vi "13.4.1 Realworld Particle.vi"(8 "ErrI":errorcluster) -> (0 "ErrO":errorcluster)   [LabVIEW 2016]
uses:
  <vilib>/vision/Image Controls.llb/IMAQ Image.ctl
  <vilib>/vision/Calibration.llb/Distortion Model.ctl
  <vilib>/vision/Calibration.llb/Distortion Model Types.ctl
  <vilib>/vision/Measure.llb/Edge Options.ctl
  <vilib>/vision/Measure.llb/Edge Polarity.ctl
  <vilib>/vision/NI_Vision_Development_Module.lvlib
panel:
  out "Center of Mass of Holes\n(mm, x and y to orign)":dbl[][](array[numeric]) format="%.2f"
  out "Image":T1(plugin-control)
  in  "Next":bool
  in  "Exit":bool
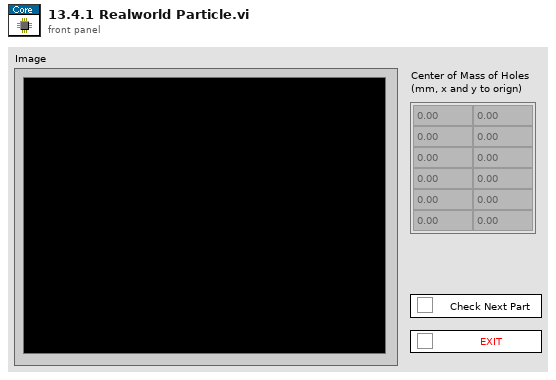
[diagram p1: front panel]
types:
  T1 = typedef "IMAQ Image.ctl" = refnum<image>
  T2 = typedef "Distortion Model.ctl" = cluster{"Distortion Model":T3, "Polynomial Model Setup":cluster{"Radial Coefficient":u32, "Tangential Coefficients ":bool}}
  T3 = typedef "Distortion Model Types.ctl" = i32
  T4 = typedef "Edge Options.ctl" = cluster{"Edge Polarity":T5, "Kernel Size":u32, "Width":u32, "Minimum Edge Strength":sgl, "Interpolation Type":enum32{"Zero Order", "Bilinear", "Quadratic", "Cubic", "Bilinear Fixed"}, "Data Processing Method":enum32{"Average", "Median"}}
  T5 = typedef "Edge Polarity.ctl" = u32
  T6 = cluster{"Direction":u16, "Primary Edge Options":T4, "Secondary Edge Options":T4, "Show Search Area":bool, "Show Search Lines":bool, "Show Edges Found":bool, "Show Result":bool, "Search Area Color":u32, "Search Lines Color":u32, "Edge Locations Color":u32, "Result Color":u32, "Overlay Group Name":string}
  T7 = typedef "IMAQ Rectangle" = cluster{"Left":i32, "Top":i32, "Right":i32, "Bottom":i32, "Rotation":dbl}
  T8 = typedef "Particle Parameters" = i32
  T9 = cluster{"Measurement Parameter":T8, "Range Lower Value":dbl, "Range Upper Value":dbl, "Range":bool, "Measurement Type":bool}[]
  T10 = cluster{"Src":T1, "Cal":T1, "Dst":T1, "Parts":string[]}
  T11 = typedef "Image Unit" = enum32{"Undefined", "Angström", "Micrometer", "Millimeter", "Centimeter", "Meter", "Kilometer", "Microinch", "Inch", "Feet", "Nautical miles", "Standard miles", "Steps"}
  T12 = typedef "Calibration Reference Points.ctl" = cluster{"Pixel Coordinates":cluster{"X":dbl, "Y":dbl}[], "Real World Coordinates":cluster{"X":dbl, "Y":dbl}[], "Unit":T11, "Image Size":cluster{"X":u32, "Y":u32}}
  T13 = typedef "ROI Descriptor" = cluster{"Global Rectangle":i32[], "Contours":cluster{"ID":enum32{"External", "Internal"}, "Type":u32, "Coordinates":i32[]}[]}
  T14 = typedef "IMAQ Coordinate System" = cluster{"Reference System":cluster{"Origin":cluster{"X":sgl, "Y":sgl}, "Angle (deg)":sgl, "Axis Reference":u32}, "Measurement System":cluster{"Origin":cluster{"X":sgl, "Y":sgl}, "Angle (deg)":sgl, "Axis Reference":u32}}
  T15 = cluster{"Origin":cluster{"X":sgl, "Y":sgl}, "Angle (deg)":sgl, "Axis Reference":u32}
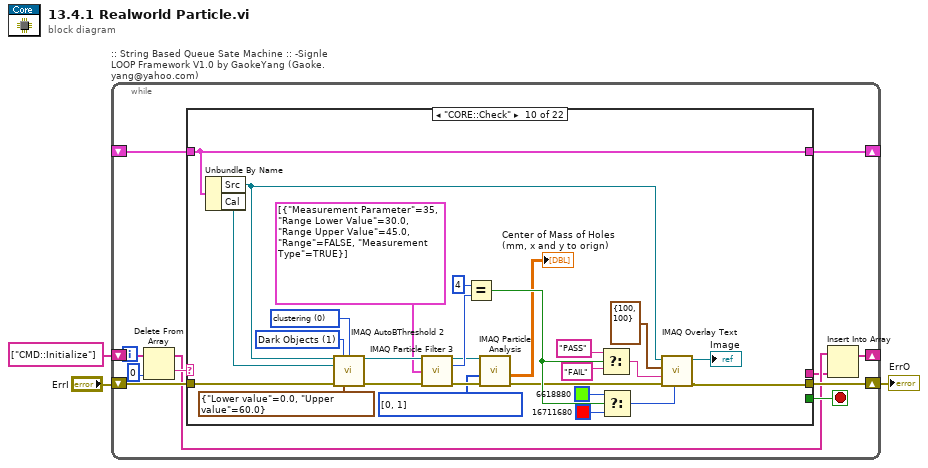
[diagram p0: block diagram]
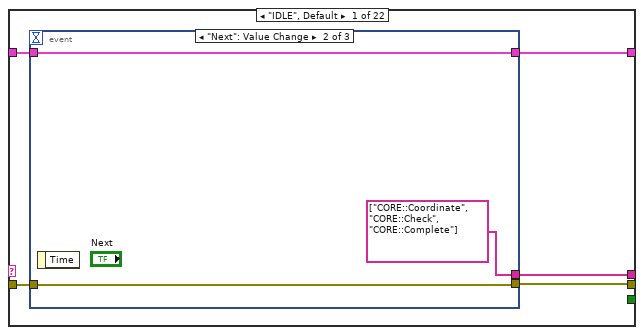
[diagram p2: hidden frame]
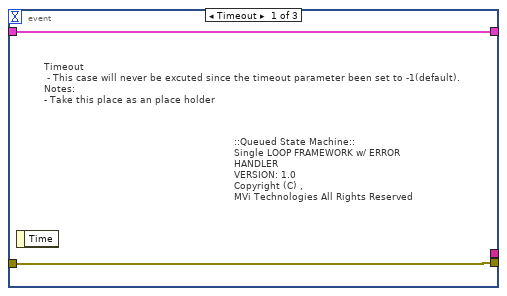
[diagram p3: hidden frame]
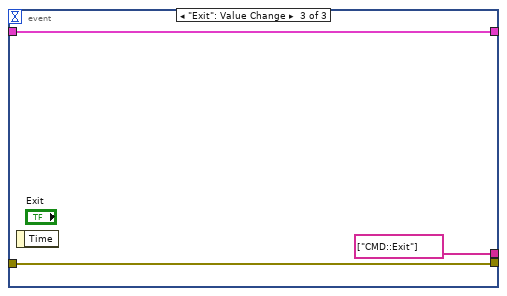
[diagram p4: hidden frame]
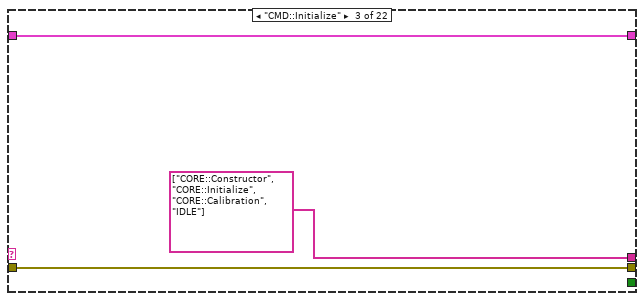
[diagram p6: hidden frame]
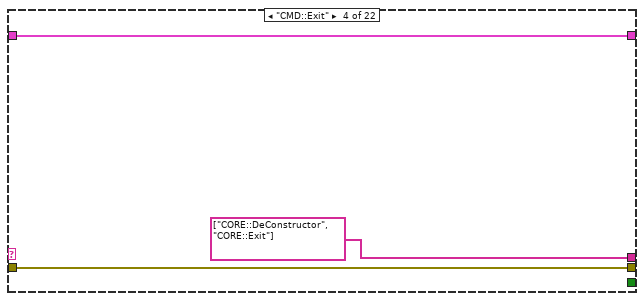
[diagram p7: hidden frame]
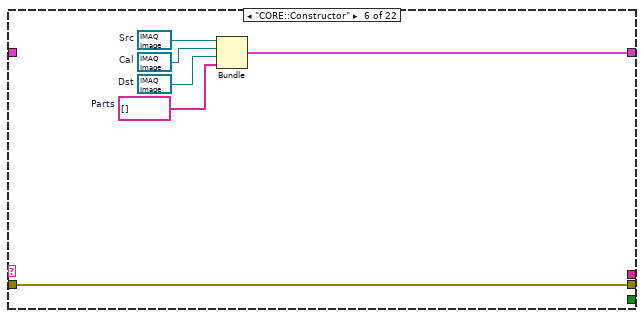
[diagram p9: hidden frame]
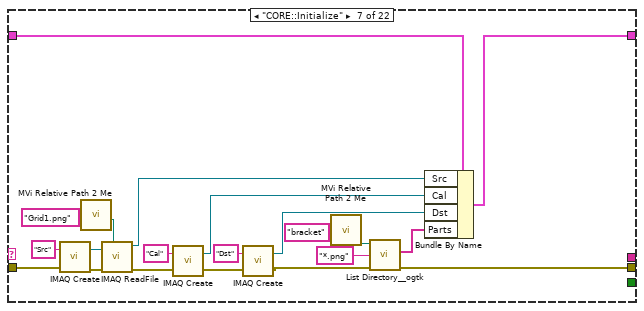
[diagram p10: hidden frame]
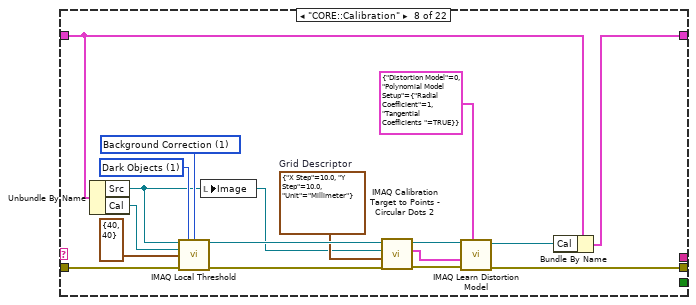
[diagram p11: hidden frame]
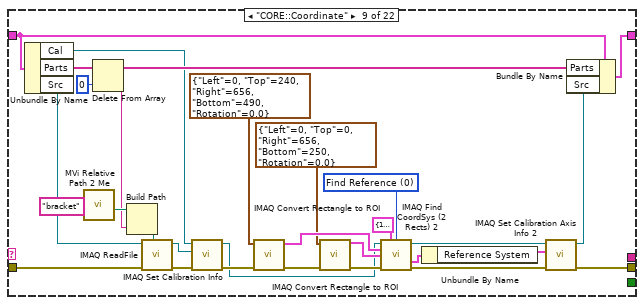
[diagram p12: hidden frame]
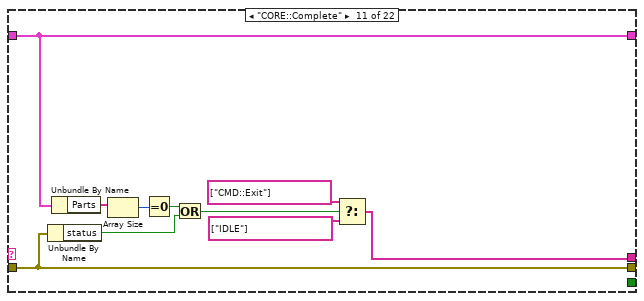
[diagram p13: hidden frame]
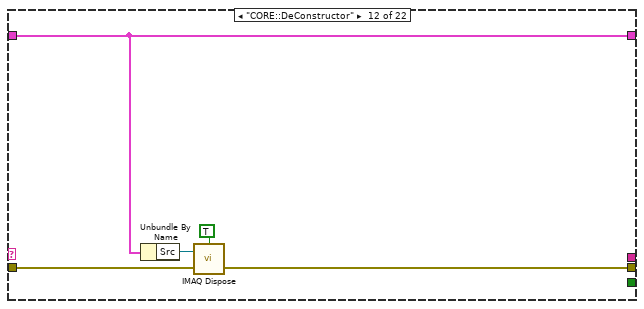
[diagram p14: hidden frame]
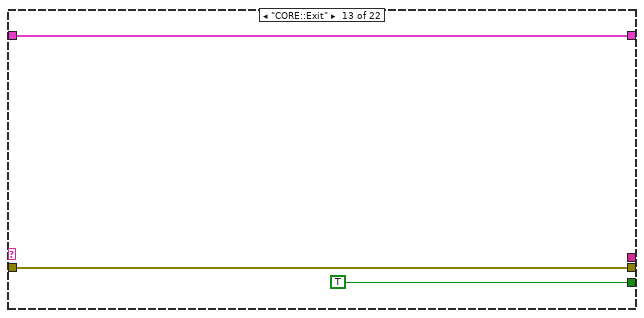
[diagram p15: hidden frame]
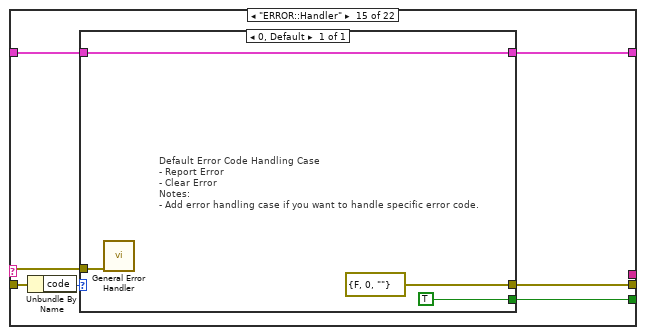
[diagram p17: hidden frame]
diagram:
  n1 = while ":: String Based Queue Sate Machine :: -Signle LOOP Framework V1.0 by GaokeYang (Gaoke.yang@yahoo.com)" {
    shift-right: [w11] -> w3
    shift-left: "ErrI" -> [w9]
    shift-right: [w13] -> _
    shift-left: _ -> [w12]
    shift-right: [w4] -> _
    shift-left: string[] ["CMD::Initialize"] -> [w10]
    stop <- w14 stop-if-true
    n2 = Delete From Array(array=w10, index=0) -> (deleted portion=w8:string, array with subset deleted=w6:string[])  [unwired: 1 in]
    n3 = case shown="\"CORE::Check\"" w8 {
      tunnel: [w18 w29 w31 w34 w37 w40 w49 w70 w85 w113 w144 w152 w154 w158 w161 w169 w171 w173 w176 w178 w180 w181] -> w11
      tunnel: [_ _ _ _ _ _ _ _ _ _ _ _ TRUE _ w160 _ _ _ _ _ _ _] -> w14
      tunnel: w9 -> [w19 w29 w31 w34 w37 w40 w56 w80 w106 w138 w144 w153 w154 w158 w159 w169 w171 w173 w176 w178 w180 w181]
      tunnel: [w16 w28 w32 w35 w36 w43 w61 w67 w100 w137 w145 w151 w155 w157 w162 w170 w172 w174 w175 w177 w179 w182] -> w13
      tunnel: w12 -> [w17 w28 w32 w35 w36 _ w62 w68 w101 w137 w145 w151 w155 w157 w163 w170 w172 w174 w175 w177 w179 w182]
      tunnel: [w15 _ string[] ["CORE::Constructor", "CORE::Initialize", "CORE::Calibration", "IDLE"] string[] ["CORE::DeConstructor", "CORE::Exit"] _ _ _ _ _ _ w146 _ _ _ _ _ _ _ _ _ _ _] -> w5
      frame "IDLE", Default {
        n4 = event shown="[1] \"Next\": Value Change" {
          selector: _ -> [_ _ _]
          dyn-events: _ -> [_ _ _]
          timeout: _ -> [_ _ _]
          tunnel: [w21 w24 w27] -> w18
          tunnel: w19 -> [w21 w24 w27]
          tunnel: [w20 w23 w26] -> w16
          tunnel: w17 -> [w20 w23 w26]
          tunnel: [_ string[] ["CORE::Coordinate", "CORE::Check", "CORE::Complete"] string[] ["CMD::Exit"]] -> w15
          event Timeout {
            # "Timeout\n - This case will never be excuted since the timeout parameter been set to -1(default).\nNotes:\n- Take this place as an place holder"
            # "::Queued State Machine::\nSingle LOOP FRAMEWORK w/ ERROR HANDLER\nVERSION: 1.0\nCopyright (C) ,\nMVi Technologies All Rights Reserved"
            n5 = event-data() -> ()  [unwired: 1 in, 1 out]
          }
          event "Next": Value Change {
            n6 = event-data() -> ()  [unwired: 1 in, 1 out]
          }
          event "Exit": Value Change {
            n7 = event-data() -> ()  [unwired: 1 in, 1 out]
          }
        }
      }
      frame "-------- Commands ---------" {
      }
      frame "CMD::Initialize" {
      }
      frame "CMD::Exit" {
      }
      frame "------------ Core ------------" {
      }
      frame "CORE::Constructor" {
        w39 = T1 refnum  # Dst
        w38 = string[] []  # Parts
        w41 = T1 refnum  # Cal
        w42 = T1 refnum  # Src
        n8 = Bundle("Src"=w42, "Cal"=w41, "Dst"=w39, "Parts"=w38) -> (w43:T10)  [unwired: 1 in]
      }
      frame "CORE::Initialize" {
        n9 = call "IMAQ Create"("Image Name"="Src", "error in (no error)"=w56) -> ("Src"=w59:T1, "error out"=w57:errorcluster)  [unwired: 3 in]
        n10 = call "MVi Relative Path 2 Me.vi"("Relative Path"="Grid1.png" ("name or relative path")) -> ("Appended Dir"=w58:path)  [unwired: 5 in, 1 out]
        n11 = call "IMAQ ReadFile"("File Path"=w58, "error in (no error)"=w57, "Image"=w59) -> ("error out"=w55:errorcluster, "Image Out"=w53:T1)  [unwired: 4 in, 3 out]
        n12 = call "IMAQ Create"("Image Name"="Cal", "error in (no error)"=w55) -> ("Src"=w54:T1, "error out"=w47:errorcluster)  [unwired: 3 in]
        n13 = call "IMAQ Create"("Image Name"="Dst", "error in (no error)"=w47) -> ("Src"=w45:T1, "error out"=w46:errorcluster)  [unwired: 3 in]
        n14 = call "MVi Relative Path 2 Me.vi"("Relative Path"="bracket" ("name or relative path")) -> ("Appended Dir"=w51:path)  [unwired: 5 in, 1 out]
        n15 = call "List Directory__ogtk.vi"("error in (no error)"=w46, "pattern"="*.png", "directory path"=w51) -> ("error out"=w49:errorcluster, "file names"=w44:string[])  [unwired: 1 in, 2 out]
        n16 = Bundle By Name(cluster=w62, "Src"=w53, "Cal"=w54, "Dst"=w45, "Parts"=w44) -> (w61:T10)
      }
      frame "CORE::Calibration" {
        w74 = cluster{"X Step":sgl, "Y Step":sgl, "Unit":T11} {"X Step"=10.0, "Y Step"=10.0, "Unit"=enum."Millimeter"}  # Grid Descriptor
        w78 = u32 1 items=["Bright Objects", "Dark Objects"] ("Look For (Bright Objects)")
        w79 = u32 1 items=["Niblack", "Background Correction", "Sauvola"] ("Method (Niblack)")
        n17 = Unbundle By Name(w68) -> ("Src"=w66:T1, "Cal"=w75:T1)
        n18 = call "IMAQ Local Threshold"("Image Src"=w66, "Look For (Bright Objects)"=w78, "Method (Niblack)"=w79, "Image Dst"=w75, "Window Size (32x32)"=cluster{"SizeX":i32, "SizeY":i32} {"SizeX"=40, "SizeY"=40}, "error in (no error)"=w80) -> ("Image Dst Out"=w77:T1, "error out"=w76:errorcluster)  [unwired: 8 in]
        n19 = local write "Image"(w66) -> ()
        n20 = call "IMAQ Calibration Target to Points - Circular Dots 2"("error in (no error)"=w76, "Grid Descriptor"=w74, "Grayscale Image"=w66, "Target Image"=w77) -> ("error out"=w71:errorcluster, "Reference Points"=w72:T12, "Target Image (dup)"=w73:T1)  [unwired: 5 in]
        n21 = call "IMAQ Learn Distortion Model"("Distortion Model Setup"=T2 {"Distortion Model"=0, "Polynomial Model Setup"={"Radial Coefficient"=1, "Tangential Coefficients "=TRUE}}, "error in (no error)"=w71, "Reference Points"=w72, "Calibration Template Image"=w73) -> ("error out"=w70:errorcluster, "Calibration Template Image Out"=w69:T1)  [unwired: 6 in]
        n22 = Bundle By Name(cluster=w68, "Cal"=w69) -> (w67:T10)
      }
      frame "CORE::Coordinate" {
        w103 = u16 0 items=["Find Reference", "Update CoordSys"] ("Mode")
        n23 = Unbundle By Name(w101) -> ("Cal"=w99:T1, "Parts"=w105:string[], "Src"=w104:T1)
        n24 = call "MVi Relative Path 2 Me.vi"("Relative Path"="bracket" ("name or relative path")) -> ("Appended Dir"=w110:path)  [unwired: 5 in, 1 out]
        n25 = Delete From Array(array=w105, index=0) -> (deleted portion=w108:string, array with subset deleted=w102:string[])  [unwired: 1 in]
        n26 = Build Path(base path=w110, name or relative path=w108) -> (appended path=w107:path)
        n27 = call "IMAQ ReadFile"("File Path"=w107, "error in (no error)"=w106, "Image"=w104) -> ("error out"=w92:errorcluster, "Image Out"=w98:T1)  [unwired: 4 in, 3 out]
        n28 = call "IMAQ Set Calibration Info"("error in (no error)"=w92, "Image Dst"=w98, "Image Src"=w99) -> ("error out"=w91:errorcluster, "Calibrated Image"=w87:T1)  [unwired: 7 in]
        n29 = call "IMAQ Convert Rectangle to ROI"("error in (no error)"=w91, "Rectangle"=T7 {"Left"=0, "Top"=240, "Right"=656, "Bottom"=490, "Rotation"=0.0}) -> ("error out"=w90:errorcluster, "ROI Descriptor"=w97:T13)  [unwired: 7 in]
        n30 = call "IMAQ Convert Rectangle to ROI"("error in (no error)"=w90, "Rectangle"=T7 {"Left"=0, "Top"=0, "Right"=656, "Bottom"=250, "Rotation"=0.0}) -> ("error out"=w89:errorcluster, "ROI Descriptor"=w96:T13)  [unwired: 7 in]
        n31 = call "IMAQ Find CoordSys (2 Rects) 2"("Image"=w87, "Options"=T6 {"Direction"=1, "Primary Edge Options"={"Edge Polarity"=0, "Kernel Size"=3, "Width"=3, "Minimum Edge Strength"=10.0, "Interpolation Type"=enum."Bilinear Fixed", "Data Processing Method"=enum."Average"}, "Secondary Edge Options"={"Edge Polarity"=0, "Kernel Size"=3, "Width"=3, "Minimum Edge Strength"=10.0, "Interpolation Type"=enum."Bilinear Fixed", "Data Processing Method"=enum."Average"}, "Show Search Area"=FALSE, "Show Search Lines"=FALSE, "Show Edges Found"=FALSE, "Show Result"=TRUE, "Search Area Color"=65280, "Search Lines Color"=255, "Edge Locations Color"=16776960, "Result Color"=16711680, "Overlay Group Name"=""}, "Mode"=w103, "Primary ROI Descriptor"=w97, "Secondary ROI Descriptor"=w96, "error in (no error)"=w89) -> ("Image Out"=w84:T1, "Coordinate System Out"=w88:T14, "error out"=w86:errorcluster)  [unwired: 5 in, 2 out]
        n32 = Unbundle By Name(w88) -> ("Reference System"=w83:T15)
        n33 = call-poly "IMAQ Set Calibration Axis Info 2"("error in (no error)"=w86, "Calibration Axis Info"=w83, "Calibration Template Image In"=w84) -> ("error out"=w85:errorcluster, "Calibration Template Image Out"=w82:T1)  [unwired: 7 in]
        n34 = Bundle By Name(cluster=w101, "Parts"=w102, "Src"=w82) -> (w100:T10)
      }
      frame "CORE::Check" {
        w115 = T8[] [0, 1] items=["Center of Mass X", "Center of Mass Y", "First Pixel X", "First Pixel Y", "Bounding Rect Left", "Bounding Rect Top", "Bounding Rect Right", "Bounding Rect Bottom", "Max Feret Diameter Start X", "Max Feret Diameter Start Y", "Max Feret Diameter End X", "Max Feret Diameter End Y", "Max Horiz. Segment Length Left", "Max Horiz. Segment Length Right", "Max Horiz. Segment Length Row", "-", "Bounding Rect Width", "Bounding Rect Height", "Bounding Rect Diagonal", "Perimeter", "Convex Hull Perimeter", "Holes' Perimeter", "Max Feret Diameter", "Equivalent Ellipse Major Axis", "Equivalent Ellipse Minor Axis", "Equivalent Ellipse Minor Axis (Feret)", "Equivalent Rect Long Side", "Equivalent Rect Short Side", "Equivalent Rect Diagonal", "Equivalent Rect Short Side (Feret)", "Average Horiz. Segment Length", "Average Vert. Segment Length", "Hydraulic Radius", "Waddel Disk Diameter", "-", "Area", "Holes' Area", "Particle & Holes' Area", "Convex Hull Area", "Image Area", "-", "Number of Holes", "Number of Horiz. Segments", "Number of Vert. Segments", "-", "Orientation", "Max Feret Diameter Orientation", "-", "% Area/Image Area", "% Area/(Particle & Holes' Area)", "Ratio of Equivalent Ellipse Axes", "Ratio of Equivalent Rect Sides", "-", "Elongation Factor", "Compactness Factor", "Heywood Circularity Factor", "Type Factor", "-", "Sum X", "Sum Y", "Sum XX", "Sum XY", "Sum YY", "Sum XXX", "Sum XXY", "Sum XYY", "Sum YYY", "-", "Moment of Inertia XX", "Moment of Inertia XY", "Moment of Inertia YY", "Moment of Inertia XXX", "Moment of Inertia XXY", "Moment of Inertia XYY", "Moment of Inertia YYY", "Norm. Moment of Inertia XX", "Norm. Moment of Inertia XY", "Norm. Moment of Inertia YY", "Norm. Moment of Inertia XXX", "Norm. Moment of Inertia XXY", "Norm. Moment of Inertia XYY", "Norm. Moment of Inertia YYY", "Hu Moment 1", "Hu Moment 2", "Hu Moment 3", "Hu Moment 4", "Hu Moment 5", "Hu Moment 6", "Hu Moment 7"] ("Real-World Measurements")
        w135 = 0 items=["clustering", "entropy", "metric", "moments", "inter-class variance"] ("Method (clustering)")
        w136 = u32 1 items=["Bright Objects", "Dark Objects"] ("Look For (Bright Objects)")
        n35 = Unbundle By Name(w137) -> ("Src"=w114:T1, "Cal"=w116:T1)
        n36 = call "IMAQ AutoBThreshold 2"("Image Src"=w114, "Look For (Bright Objects)"=w136, "Method (clustering)"=w135, "Image Dst"=w116, "error in (no error)"=w138, "Threshold Limits"=cluster{"Lower value":sgl, "Upper value":sgl} {"Lower value"=0.0, "Upper value"=60.0}) -> ("Image Dst Out"=w132:T1, "error out"=w133:errorcluster)  [unwired: 7 in, 1 out]
        n37 = call "IMAQ Particle Filter 3"("Image Src"=w132, "Selection Values"=T9 [{"Measurement Parameter"=35, "Range Lower Value"=30.0, "Range Upper Value"=45.0, "Range"=FALSE, "Measurement Type"=TRUE}], "error in (no error)"=w133) -> ("Image Dst Out"=w118:T1, "Number of Particles"=w130:i32, "error out"=w120:errorcluster)  [unwired: 10 in]
        n38 = Equal?(x=4, y=w130) -> (x = y?=w125:bool)
        n39 = call "IMAQ Particle Analysis"("error in (no error)"=w120, "Real-World Measurements"=w115, "Image"=w118) -> ("error out"=w119:errorcluster, "Particle Measurements (Real-World)"=→"Center of Mass of Holes\n(mm, x and y to orign)":dbl[][])  [unwired: 3 in, 4 out]
        n40 = Select(t="PASS" ("String"), s=w125, f="FAIL" ("String")) -> (s? t:f=w126:string)
        n41 = Select(t=u32 6618880 ("Text Color (black)"), s=w125, f=u32 16711680 ("Text Color (black)")) -> (s? t:f=w122:u32)
        n42 = call "IMAQ Overlay Text"("Text Color (black)"=w122, "error in (no error)"=w119, "String"=w126, "Origin"=cluster{"X":i32, "Y":i32} {"X"=100, "Y"=100}, "Image"=w114) -> ("error out"=w113:errorcluster, "Image Out"=→"Image":T1)  [unwired: 5 in]
      }
      frame "CORE::Complete" {
        n43 = Unbundle By Name(w144) -> ("status"=w140:bool)
        n44 = Unbundle By Name(w145) -> ("Parts"=w143:string[])
        n45 = Array Size(array=w143) -> (size(s)=w142:i32)
        n46 = Equal To 0?(x=w142) -> (x = 0?=w141:bool)
        n47 = Or(x=w141, y=w140) -> (x .or. y?=w139:bool)
        n48 = Select(t=string[] ["CMD::Exit"], s=w139, f=string[] ["IDLE"]) -> (s? t:f=w146:string[])
      }
      frame "CORE::DeConstructor" {
        n49 = Unbundle By Name(w151) -> ("Src"=w150:T1)
        n50 = call "IMAQ Dispose"("All Images? (No)"=TRUE, "Image"=w150, "error in (no error)"=w153) -> ("error out"=w152:errorcluster)  [unwired: 3 in]
      }
      frame "CORE::Exit" {
      }
      frame "-------- Error Handle--------" {
      }
      frame "ERROR::Handler" {
        n51 = Unbundle By Name(w159) -> ("code"=w164:i32)
        n52 = case shown="0, Default" w164 {
          tunnel: [w168] -> w162
          tunnel: w163 -> [w168]
          tunnel: [errorcluster {"status"=FALSE, "code"=0, "source"=""} ("error out")] -> w161
          tunnel: [TRUE] -> w160
          tunnel: w159 -> [w166]
          frame 0, Default {
            # "Default Error Code Handling Case\n- Report Error\n- Clear Error \nNotes:\n- Add error handling case if you want to handle specific error code."
            n53 = call <vilib>:"General Error Handler.vi"("error in (no error)"=w166) -> ()  [unwired: 10 in, 5 out]
          }
        }
      }
      frame "------------  GUI  ------------" {
      }
      frame "GUI::Initialize" {
      }
      frame "GUI::SetCusor" {
      }
      frame "GUI::SetMenu" {
      }
      frame "------------ USER -----------" {
      }
      frame "USER::Case1" {
      }
      frame "USER::Case2" {
      }
    }
    n54 = Insert Into Array(array=w6, new element=w5) -> (w4:string[])  [unwired: 1 in]
  }
  "ErrO" <- w3
